vi "Read Depth Low Resolution Dani.vi"(8 "error in (no error)":errorcluster, 10 "depth":u16[](array[numeric]), 11 "Image In":T1) -> (0 "error out":errorcluster, 3 "Image Out":T1)   [LabVIEW 2015]
uses:
  <vilib>/vision/Image Controls.llb/IMAQ Image.ctl
  libkinect_wrapper.dll
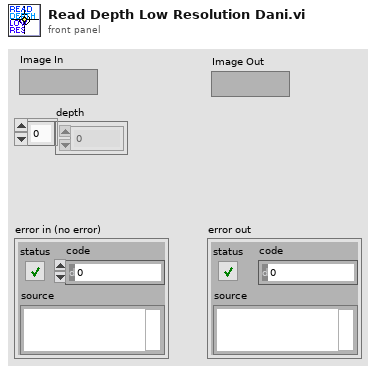
[diagram p1: front panel]
types:
  T1 = typedef "IMAQ Image.ctl" = refnum<image>
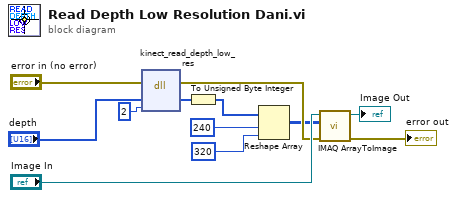
[diagram p0: block diagram]
diagram:
  n1 = dll-call lib="libkinect_wrapper.*" fn="kinect_read_depth_low_res"(error in="error in (no error)", "depth"="depth", "factor"=2) -> (error out=w7:errorcluster, "depth"=w5:u16[])  [unwired: 4 in, 1 out]
  n2 = To Unsigned Byte Integer(number=w5) -> (unsigned 8bit integer=w4:u8[])
  n3 = Reshape Array(w4, 240 ("dimension size"), 320 ("dimension size")) -> (w3:u8[][])
  n4 = call "IMAQ ArrayToImage"("error in (no error)"=w7, "Image Pixels (U8)"=w3, "Image"="Image In") -> ("error out"=→"error out":errorcluster, "Image Out"=→"Image Out":T1)  [unwired: 7 in]
